vi "Send Output Command.vi"(0 "VISA resource name":refnum<visa-resource-name>, 1 "Address (1)":u16=1 max=15 step=1, 5 "Handshake Dispense (0:None)":u16(ring) items=["None", "#1 ", "#2", "#3"], 7 "Enable Parallel Output 1":bool, 9 "Enable Parallel Output 2":bool, 11 "error in (no error)":errorcluster, 12 "Enable Parallel Output 3":bool, 13 "Serial Bits of Byte #1 of Serial Expansion Port\n                     1            2            3             4            5             6            7            8":bool[](array[boolean]), 14 "Serial Bits of Byte #2 of Serial Expansion Port\n                     1             2            3            4            5             6            7            8":bool[](array[boolean])) -> (4 "VISA resource name out":refnum<visa-resource-name>, 15 "error out":errorcluster)   [LabVIEW 2021, in "Copy of Kloehn V6 Series.lvlib"]
doc: "Utilizes the I/O on the back of the instrument. This could have many uses. There is the possibility of using the pump as a master device connected by other slave devices. There is also the possibility of handshaking or coordinating pump actions between more than one pump. Another use could involve solenoid valves."
uses:
  Copy of Kloehn V6 Series.lvlib
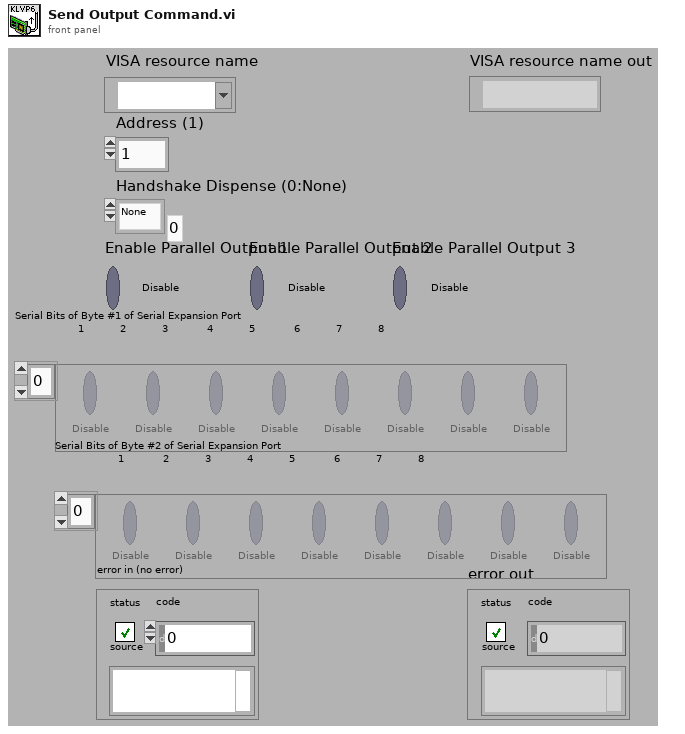
[diagram p1: front panel]
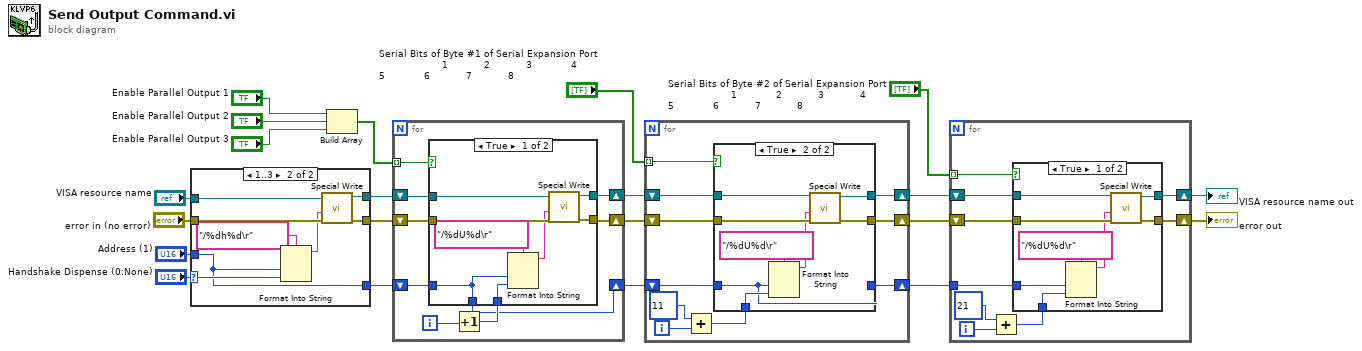
[diagram p0: block diagram]
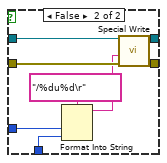
[diagram p2: hidden frame]
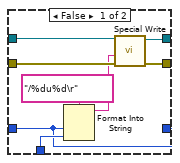
[diagram p3: hidden frame]
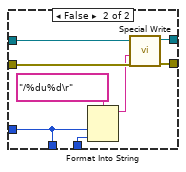
[diagram p4: hidden frame]
diagram:
  n1 = case shown="1..3" "Handshake Dispense (0:None)" {
    selector: "Handshake Dispense (0:None)" -> [_ w29]
    tunnel: "VISA resource name" -> [w24 w32]
    tunnel: "error in (no error)" -> [w23 w31]
    tunnel: "Address (1)" -> [w22 w25]
    tunnel: [w24 w27] -> w17
    tunnel: [w23 w26] -> w16
    tunnel: [w22 w25] -> w15
    frame 0, Default {
    }
    frame 1..3 {
      n2 = Format Into String(format string="/%dh%d\r", w25, w29) -> (resulting string=w28:string)  [unwired: 2 in, 1 out]
      n3 = call "Special Write.vi"("error in (no error)"=w31, "Send String"=w28, "VISA resource name"=w32) -> ("error out"=w26:errorcluster, "VISA resource name out"=w27:refnum<visa-resource-name>)  [unwired: 4 in, 3 out]
    }
  }
  n4 = Build Array("Enable Parallel Output 1", "Enable Parallel Output 2", "Enable Parallel Output 3") -> (w3:bool[])
  n5 = for {
    tunnel: w3 -> [w39] mode=indexing
    shift-right: [w34] -> w11
    shift-left: w16 -> [w37]
    shift-right: [w35] -> w12
    shift-left: w17 -> [w38]
    shift-right: [w33] -> w14
    shift-left: w15 -> [w36]
    i -> [w41]
    n6 = Increment(x=w41) -> (x+1=w40:i32)
    n7 = case shown="True" w39 {
      tunnel: w40 -> [w49 w57]
      tunnel: w38 -> [w47 w55]
      tunnel: w37 -> [w46 w54]
      tunnel: w36 -> [w42 w50]
      tunnel: [w44 w52] -> w34
      tunnel: [w43 w51] -> w35
      tunnel: [w42 w50] -> w33
      frame True {
        n8 = Format Into String(format string="/%dU%d\r", w42, w49) -> (resulting string=w45:string)  [unwired: 2 in, 1 out]
        n9 = call "Special Write.vi"("error in (no error)"=w46, "Send String"=w45, "VISA resource name"=w47) -> ("error out"=w44:errorcluster, "VISA resource name out"=w43:refnum<visa-resource-name>)  [unwired: 4 in, 3 out]
      }
      frame False {
        n10 = Format Into String(format string="/%du%d\r", w50, w57) -> (resulting string=w53:string)  [unwired: 2 in, 1 out]
        n11 = call "Special Write.vi"("error in (no error)"=w54, "Send String"=w53, "VISA resource name"=w55) -> ("error out"=w52:errorcluster, "VISA resource name out"=w51:refnum<visa-resource-name>)  [unwired: 4 in, 3 out]
      }
    }
  }
  n12 = for {
    shift-right: [w61] -> w1
    shift-left: w11 -> [w64]
    shift-right: [w62] -> w2
    shift-left: w12 -> [w65]
    tunnel: "Serial Bits of Byte #1 of Serial Expansion Port\n                     1            2            3             4            5             6            7            8" -> [w60] mode=indexing
    shift-right: [w59] -> w10
    shift-left: w14 -> [w63]
    i -> [w67]
    n13 = Add(x=11, y=w67) -> (x+y=w66:i32)
    n14 = case shown="True" w60 {
      tunnel: w66 -> [w75 w83]
      tunnel: w65 -> [w73 w81]
      tunnel: w64 -> [w72 w80]
      tunnel: w63 -> [w68 w76]
      tunnel: [w70 w78] -> w61
      tunnel: [w69 w77] -> w62
      tunnel: [w68 w76] -> w59
      frame False {
        n15 = Format Into String(format string="/%du%d\r", w68, w75) -> (resulting string=w71:string)  [unwired: 2 in, 1 out]
        n16 = call "Special Write.vi"("error in (no error)"=w72, "Send String"=w71, "VISA resource name"=w73) -> ("error out"=w70:errorcluster, "VISA resource name out"=w69:refnum<visa-resource-name>)  [unwired: 4 in, 3 out]
      }
      frame True {
        n17 = Format Into String(format string="/%dU%d\r", w76, w83) -> (resulting string=w79:string)  [unwired: 2 in, 1 out]
        n18 = call "Special Write.vi"("error in (no error)"=w80, "Send String"=w79, "VISA resource name"=w81) -> ("error out"=w78:errorcluster, "VISA resource name out"=w77:refnum<visa-resource-name>)  [unwired: 4 in, 3 out]
      }
    }
  }
  n19 = for {
    tunnel: w10 -> [w88]
    shift-right: [w86] -> w7
    shift-left: w1 -> [w89]
    shift-right: [w87] -> w8
    shift-left: w2 -> [w90]
    tunnel: "Serial Bits of Byte #2 of Serial Expansion Port\n                     1             2            3            4            5             6            7            8" -> [w85] mode=indexing
    i -> [w92]
    n20 = Add(x=21, y=w92) -> (x+y=w91:i32)
    n21 = case shown="True" w85 {
      tunnel: w91 -> [w100 w108]
      tunnel: w90 -> [w97 w105]
      tunnel: w89 -> [w96 w104]
      tunnel: w88 -> [w99 w107]
      tunnel: [w94 w102] -> w86
      tunnel: [w93 w101] -> w87
      frame True {
        n22 = Format Into String(format string="/%dU%d\r", w99, w100) -> (resulting string=w95:string)  [unwired: 2 in, 1 out]
        n23 = call "Special Write.vi"("error in (no error)"=w96, "Send String"=w95, "VISA resource name"=w97) -> ("error out"=w94:errorcluster, "VISA resource name out"=w93:refnum<visa-resource-name>)  [unwired: 4 in, 3 out]
      }
      frame False {
        n24 = Format Into String(format string="/%du%d\r", w107, w108) -> (resulting string=w103:string)  [unwired: 2 in, 1 out]
        n25 = call "Special Write.vi"("error in (no error)"=w104, "Send String"=w103, "VISA resource name"=w105) -> ("error out"=w102:errorcluster, "VISA resource name out"=w101:refnum<visa-resource-name>)  [unwired: 4 in, 3 out]
      }
    }
  }
  "VISA resource name out" <- w8
  "error out" <- w7
